vi "Filter Isolated Endpoints.vi"(11 "Possible Connections in":T2(array[cluster])) -> (3 "Possible Connections out":T2(array[cluster]))   [LabVIEW 2017, in "Routing and Faulting System Explorer.lvlib"]
uses:
  Routing and Faulting System Explorer.lvlib
  Shared/Routing and Faulting Hardware API/Types/Possible Connections for Endpoint.ctl
  Shared/Routing and Faulting Hardware API/Routing and Faulting Hardware API.lvlib
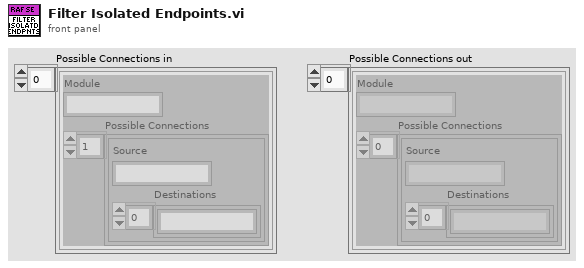
[diagram p1: front panel]
types:
  T1 = typedef "Routing and Faulting Hardware API.lvlib/Possible Connections for Endpoint.ctl" = cluster{"Source":string, "Destinations":string[]}
  T2 = cluster{"Module":string, "Possible Connections":T1[]}[]
  T3 = cluster{"Module":string, "Possible Connections":T1[]}
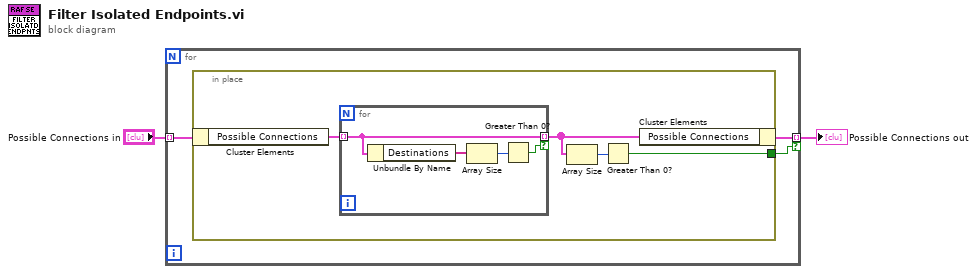
[diagram p0: block diagram]
diagram:
  n1 = for {
    tunnel: "Possible Connections in" -> [w5] mode=indexing
    tunnel: [w4] -> w1 mode=indexing if=w3
    n2 = in-place {
      in-place-border: [w6] -> w3
      n3 = in-place-cluster #1(w5) -> ("Possible Connections"=w9:T1[])
      n4 = for {
        tunnel: w9 -> [w11] mode=indexing
        tunnel: [w11] -> w7 mode=indexing if=w10
        n5 = Unbundle By Name(w11) -> ("Destinations"=w13:string[])
        n6 = Array Size(array=w13) -> (size(s)=w12:i32)
        n7 = Greater Than 0?(x=w12) -> (x > 0?=w10:bool)
      }
      n8 = Array Size(array=w7) -> (size(s)=w8:i32)
      n9 = Greater Than 0?(x=w8) -> (x > 0?=w6:bool)
      n10 = in-place-cluster #1("Possible Connections"=w7) -> (w4:T3)
    }
  }
  "Possible Connections out" <- w1
